vi "Thermocouple 4353 .vi"(11 "Temp Convergence Criteria [deg C]":dbl=0.01 min=0.0 max=200.0 step=0.01 format="%#.2f") -> (3 "Temperature Data":dbl[](array[numeric]))   [LabVIEW 2021]
uses:
  <vilib>/DAQmx/read.llb/DAQmx Read (Analog 2D DBL NChan NSamp).vi
  <vilib>/DAQmx/create/channels.llb/DAQmx Create Channel (AI-Temperature-Thermocouple).vi
  <vilib>/DAQmx/configure/timing.llb/DAQmx Timing (Sample Clock).vi
  <vilib>/DAQmx/miscellaneous.llb/DAQmx Fill In Error Info.vi
  <resource>/objmgr/daqmx.rc
panel:
  out "Themocouple Probes":T1 {"32" format="%#.2f"; "31" format="%#.2f"; "30" format="%#.2f"; "29" format="%#.2f"; "28" format="%#.2f"; "27" format="%#.2f"; "26" format="%#.2f"; "25" format="%#.2f"; "24" format="%#.2f"; "23" format="%#.2f"; "22" format="%#.2f"; "21" format="%#.2f"; "20" format="%#.2f"; "19" format="%#.2f"; "18" format="%#.2f"; "17" format="%#.2f"; "16" format="%#.2f"; "15" format="%#.2f"; "14" format="%#.2f"; "13" format="%#.2f"; "12" format="%#.2f"; "11" format="%#.2f"; "10" format="%#.2f"; "9" format="%#.2f"; "8" format="%#.2f"; "7" format="%#.2f"; "6" format="%#.2f"; "5" format="%#.2f"; "4" format="%#.2f"; "3" format="%#.2f"; "2" format="%#.2f"; "1" format="%#.2f"}
  out "Elapsed Time":u16 caption="Test Countdown [Seconds]" format="%#.0f"
  in  "Read Delay [Seconds]":dbl=30.0
  out "Temperature Deltas":dbl[](graph)
  in  "Physical Channel":tag="PXIe-4353/ai0:31"
  in  "Abort":bool
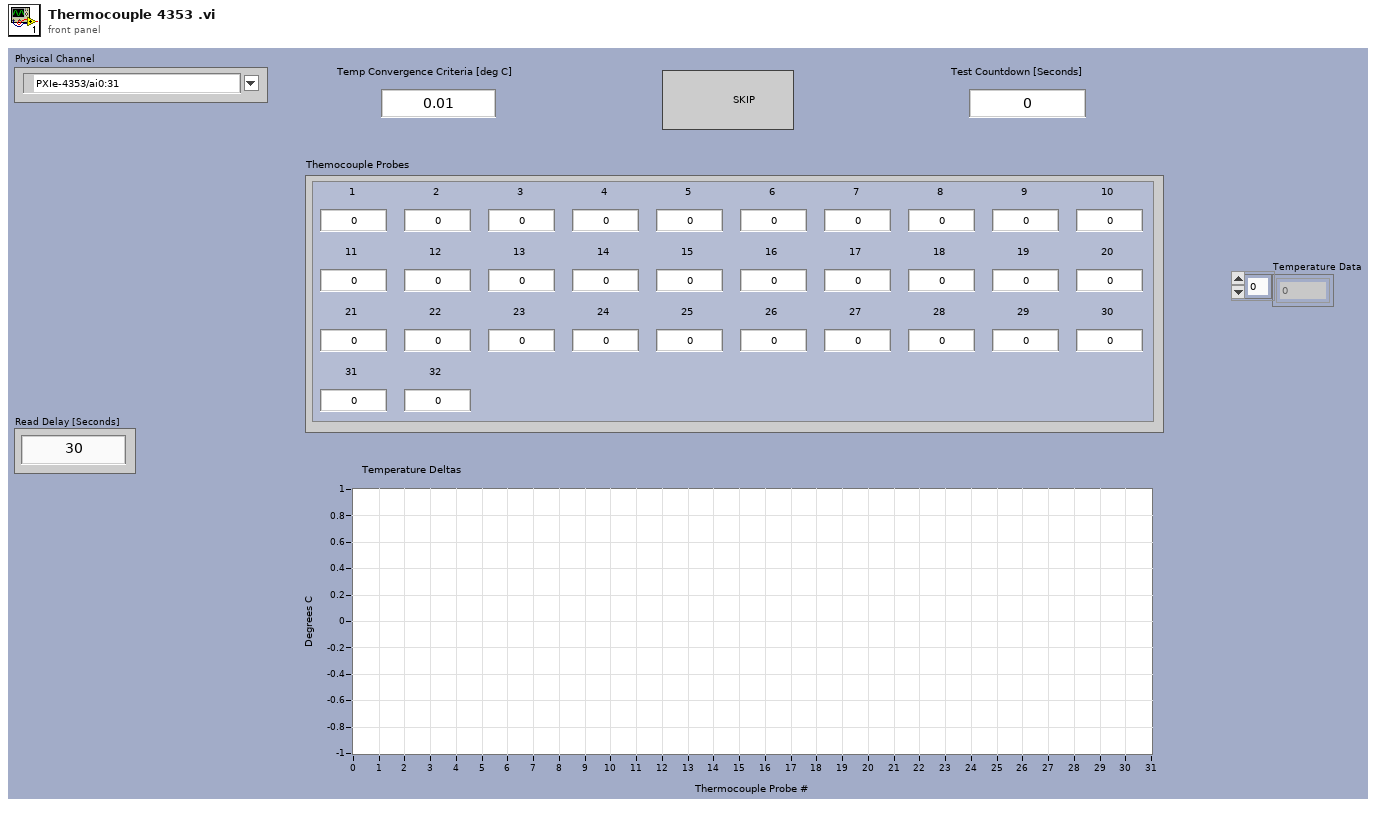
[diagram p1: front panel]
types:
  T1 = cluster{"1":dbl, "2":dbl, "3":dbl, "4":dbl, "5":dbl, "6":dbl, "7":dbl, "8":dbl, "9":dbl, "10":dbl, "11":dbl, "12":dbl, "13":dbl, "14":dbl, "15":dbl, "16":dbl, "17":dbl, "18":dbl, "19":dbl, "20":dbl, "21":dbl, "22":dbl, "23":dbl, "24":dbl, "25":dbl, "26":dbl, "27":dbl, "28":dbl, "29":dbl, "30":dbl, "31":dbl, "32":dbl}
  T2 = cluster{"[0]":dbl, "[1]":dbl, "[2]":dbl, "[3]":dbl, "[4]":dbl, "[5]":dbl, "[6]":dbl, "[7]":dbl, "[8]":dbl, "[9]":dbl, "[10]":dbl, "[11]":dbl, "[12]":dbl, "[13]":dbl, "[14]":dbl, "[15]":dbl, "[16]":dbl, "[17]":dbl, "[18]":dbl, "[19]":dbl, "[20]":dbl, "[21]":dbl, "[22]":dbl, "[23]":dbl, "[24]":dbl, "[25]":dbl, "[26]":dbl, "[27]":dbl, "[28]":dbl, "[29]":dbl, "[30]":dbl, "[31]":dbl}
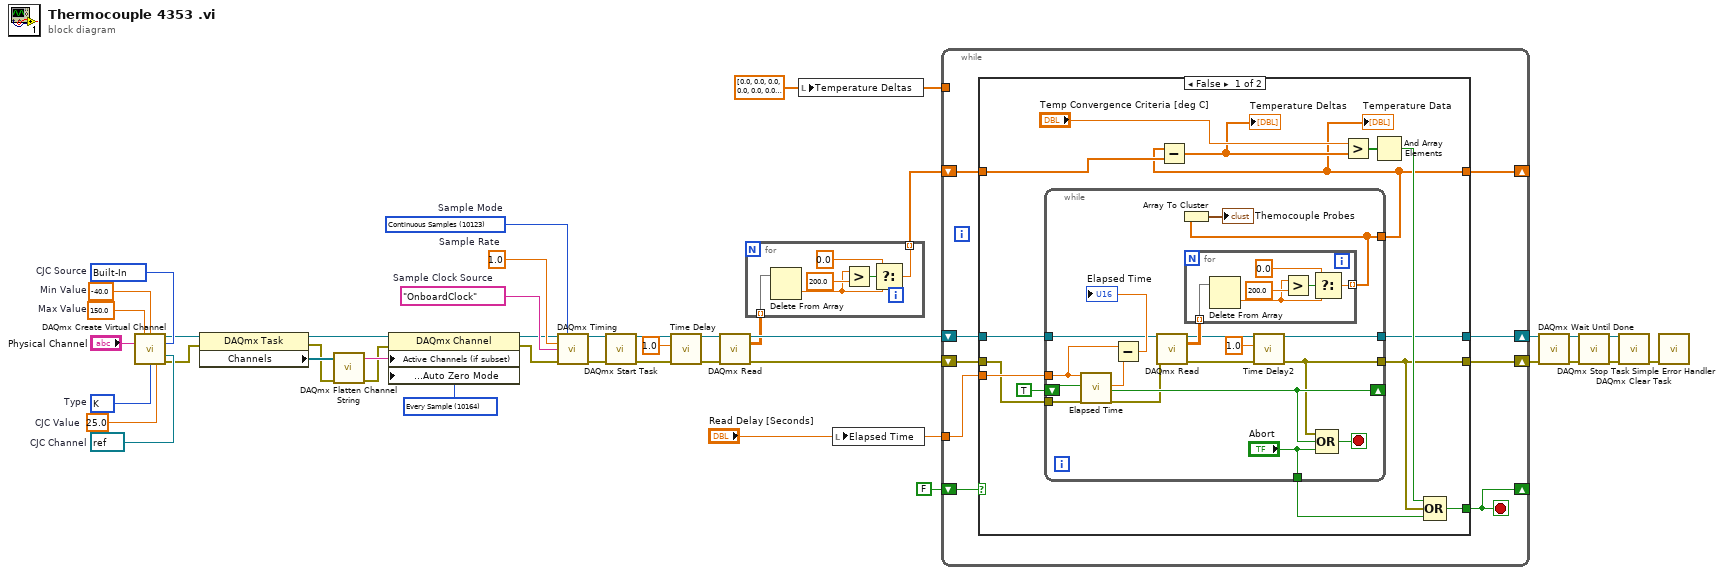
[diagram p0: block diagram]
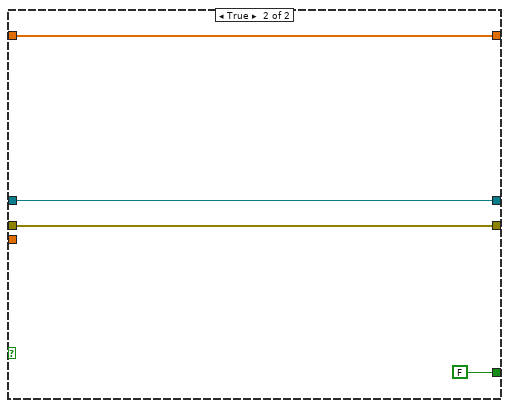
[diagram p2: hidden frame]
diagram:
  w8 = 10164 items=["None"=10230, "Once"=10244, "Every Sample"=10164] ("Auto Zero Mode")
  w7 = dbl[] [0.0, 0.0, 0.0, 0.0, 0.0, 0.0, 0.0, 0.0, 0.0, 0.0, 0.0, 0.0, 0.0, 0.0, 0.0, 0.0, 0.0, 0.0, 0.0, 0.0, 0.0, 0.0, 0.0, 0.0, 0.0, 0.0, 0.0, 0.0, 0.0, 0.0, 0.0, 0.0]
  w39 = refnum<k21> refnum  # CJC Channel
  w34 = 10200 items=["Built-In"=10200, "Constant Value"=10116, "Channel"=10113]  # CJC Source
  w35 = -40.0  # Min Value
  w36 = 150.0  # Max Value
  w38 = 25.0  # CJC Value
  w37 = 10073 items=["J"=10072, "K"=10073, "N"=10077, "R"=10082, "S"=10085, "T"=10086, "B"=10047, "E"=10055]  # Type
  w30 = 1.0  # Sample Rate
  w31 = tag "OnboardClock"  # Sample Clock Source
  w33 = 10123 items=["Finite Samples"=10178, "Continuous Samples"=10123, "Hardware Timed Single Point"=12522]  # Sample Mode
  n1 = call-poly <vilib>:"DAQmx Create Virtual Channel.vi"("maximum value"=w36, "minimum value"=w35, "physical channels"="Physical Channel", "cjc source"=w34, "cjc channel"=w39, "thermocouple type"=w37, "cjc value"=w38) -> ("task out"=w17:refnum<k21>, "error out"=w15:errorcluster)  [unwired: 7 in]
  n2 = property class="DAQmx Task"(reference=w17, error in=w15) -> (reference out=w13:refnum<k21>, error out=w10:errorcluster, "Channels"=w12:refnum<k21>[])
  n3 = call <vilib>:"DAQmx Flatten Channel String.vi"("names in"=w12, "error in"=w10) -> ("names out"=w11:string, "error out"=w9:errorcluster)  [unwired: 12 in]
  n4 = property class="DAQmx Channel"(reference=w13, error in=w9, "Active Channels (if subset)"=w11, "Analog Input:General Properties:Advanced:High Accuracy Settings:Auto Zero Mode"=w8) -> (reference out=w16:refnum<k21>, error out=w14:errorcluster)
  n5 = call-poly <vilib>:"DAQmx Timing.vi"("task/channels in"=w16, "sample mode"=w33, "rate"=w30, "source"=w31, "error in"=w14) -> ("task out"=w28:refnum<k21>, "error out"=w29:errorcluster)  [unwired: 9 in]
  n6 = call <vilib>:"DAQmx Start Task.vi"("task/channels in"=w28, "error in"=w29) -> ("task out"=w20:refnum<k21>, "error out"=w23:errorcluster)  [unwired: 12 in]
  n7 = call "Time Delay"("error in (no error)"=w23, "Delay Time (s)"=1.0) -> ("error out"=w21:errorcluster)  [unwired: 9 in]
  n8 = call-poly <vilib>:"DAQmx Read.vi"("task/channels in"=w20, "error in"=w21) -> ("task out"=w19:refnum<k21>, "data"=w6:dbl[][], "error out"=w18:errorcluster)  [unwired: 11 in]
  n9 = for {
    tunnel: [w43] -> w5 mode=indexing
    tunnel: w6 -> [w41] mode=indexing
    n10 = Delete From Array(array=w41) -> (deleted portion=w42:dbl)  [unwired: 2 in, 1 out]
    n11 = Greater?(x=w42, y=200.0) -> (0:w45:bool)
    n12 = Select(t=0.0, s=w45, f=w42) -> (s? t:f=w43:dbl)
  }
  n13 = local write "Temperature Deltas"(w7) -> ()
  n14 = local write "Elapsed Time"("Read Delay [Seconds]") -> ()
  n15 = while {
    shift-right: [w47] -> _
    shift-left: w5 -> [w55]
    shift-right: [w54] -> _
    shift-left: FALSE -> [w53]
    tunnel: "Read Delay [Seconds]" -> [w52]
    shift-right: [w50] -> w4
    shift-left: w19 -> [w49]
    shift-right: [w51] -> w2
    shift-left: w18 -> [w48]
    tunnel: w7 -> [_]
    stop <- w54 stop-if-true
    n16 = case shown="False" w53 {
      tunnel: [w62 FALSE] -> w54
      tunnel: w55 -> [w67 w96]
      tunnel: [w56 w96] -> w47
      tunnel: w48 -> [w61 w93]
      tunnel: w49 -> [w60 w94]
      tunnel: w52 -> [w65 _]
      tunnel: [w59 w94] -> w50
      tunnel: [w58 w93] -> w51
      frame False {
        n17 = while {
          tunnel: w65 -> [w81]
          shift-right: [w83] -> _
          shift-left: TRUE ("Time has Elapsed") -> [w86]
          tunnel: w61 -> [w85]
          tunnel: ["Abort"] -> w63
          tunnel: [w70] -> w58
          tunnel: w60 -> [w76]
          tunnel: [w75] -> w59
          tunnel: [w73] -> w56
          stop <- w84 stop-if-true
          n18 = call "Elapsed Time"("Time Target (s)"=w81, "Reset"=w86, "error in (no error)"=w85) -> ("Elapsed Time (s)"=w79:dbl, "Time has Elapsed"=w83:bool, "error out"=w77:errorcluster)  [unwired: 9 in, 5 out]
          n19 = Subtract(x=w81, y=w79) -> (x-y=→"Elapsed Time":dbl)
          n20 = call-poly <vilib>:"DAQmx Read.vi"("task/channels in"=w76, "error in"=w77) -> ("task out"=w75:refnum<k21>, "data"=w78:dbl[][], "error out"=w71:errorcluster)  [unwired: 11 in]
          n21 = for {
            tunnel: w78 -> [w88] mode=indexing
            tunnel: [w87] -> w73 mode=indexing
            n22 = Delete From Array(array=w88) -> (deleted portion=w89:dbl)  [unwired: 2 in, 1 out]
            n23 = Greater?(x=w89, y=200.0) -> (0:w91:bool)
            n24 = Select(t=0.0, s=w91, f=w89) -> (s? t:f=w87:dbl)
          }
          n25 = Array To Cluster(array=w73) -> (cluster=→"Themocouple Probes":T2)
          n26 = call "Time Delay2"("error in (no error)"=w71, "Delay Time (s)"=1.0) -> ("error out"=w70:errorcluster)  [unwired: 9 in]
          n27 = Compound Arithmetic op=OR(w70, w83, "Abort") -> (w84:bool)
        }
        "Temperature Data" <- w56
        n28 = Subtract(x=w56, y=w67) -> (x-y=w57:dbl[])
        "Temperature Deltas" <- w57
        n29 = Greater?(x="Temp Convergence Criteria [deg C]", y=w57) -> (0:w69:bool[])
        n30 = And Array Elements(Boolean array=w69) -> (logical AND=w68:bool)
        n31 = Compound Arithmetic op=OR(w68, w58, w63) -> (w62:bool)
      }
      frame True {
      }
    }
  }
  n32 = call <vilib>:"DAQmx Wait Until Done.vi"("task/channels in"=w4, "error in"=w2) -> ("task out"=w3:refnum<k21>, "error out"=w1:errorcluster)  [unwired: 12 in]
  n33 = call <vilib>:"DAQmx Stop Task.vi"("task/channels in"=w3, "error in"=w1) -> ("task out"=w27:refnum<k21>, "error out"=w26:errorcluster)  [unwired: 12 in]
  n34 = call <vilib>:"DAQmx Clear Task.vi"("task in"=w27, "error in"=w26) -> ("error out"=w25:errorcluster)  [unwired: 13 in]
  n35 = call <vilib>:"Simple Error Handler.vi"("error in (no error)"=w25) -> ()  [unwired: 4 in, 5 out]
